vi "Example XYGraph Cursors.vi"() -> ()   [LabVIEW 2020]
uses:
  controls/CursorOptions.ctl
  Graph Extensions.lvlib
  <vilib>/ptbypt/NI_PtbyPt.lvlib
panel:
  in  "Cursor Options":T1={"font"={"Font Name"="Arial", "Size"=15, "Strikeout?"=FALSE, "Italic?"=FALSE, "Underline?"=FALSE, "Outline?"=FALSE, "Shadow?"=FALSE, "Bold?"=FALSE}, "size"=2, "Timestamp"=enum."at BOTTOM", "Vertical Line?"=TRUE, "Horizontal Line?"=TRUE, "alignment(left, top)"={"horizontal"=enum."left", "vertical"=enum."center"}, "TextFormat"=" %3$s\\n %2$.2f", "time format (%H:%M:%S)"="%I:%M:%S %p"} {"size" min=1 max=50}
  out "XY Graph":cluster{dbl[], dbl[]}[](graph)
  # "Instructions: Move the mouse over the graphs, and adjust any of the options at the right. to see the effect."
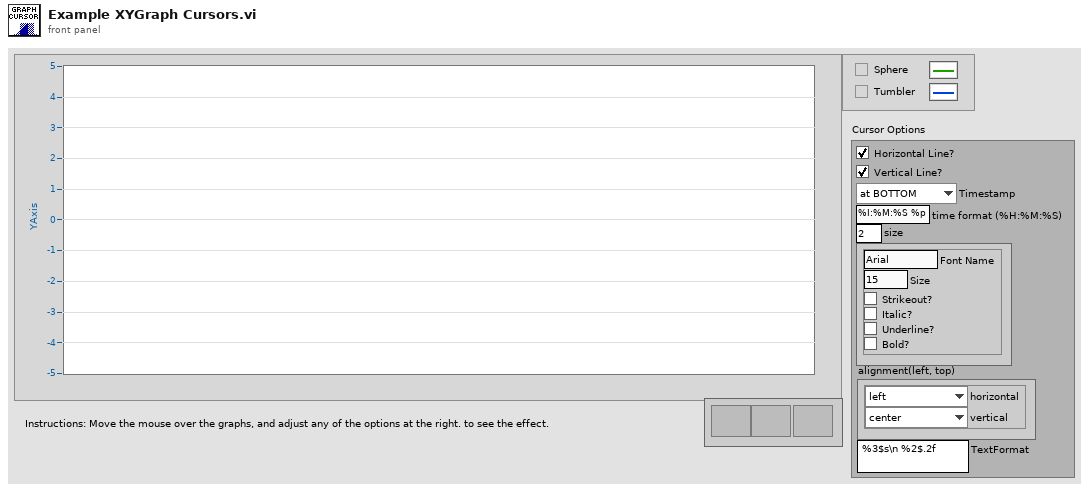
[diagram p1: front panel]
types:
  T1 = typedef "Graph Extensions.lvlib/CursorOptions.ctl" = cluster{"font":cluster{"Font Name":string, "Size":i16, "Strikeout?":bool, "Italic?":bool, "Underline?":bool, "Outline?":bool, "Shadow?":bool, "Bold?":bool}, "size":i16, "Timestamp":enum16{"at TOP", "at BOTTOM", "none"}, "Vertical Line?":bool, "Horizontal Line?":bool, "alignment(left, top)":cluster{"horizontal":enum16{"left", "center", "right"}, "vertical":enum16{"top", "center", "bottom"}}, "TextFormat":string, "time format (%H:%M:%S)":string}
  T2 = typedef "LVPoint32TypeDef.ctl" = cluster{"Horizontal":i32, "Vertical":i32}
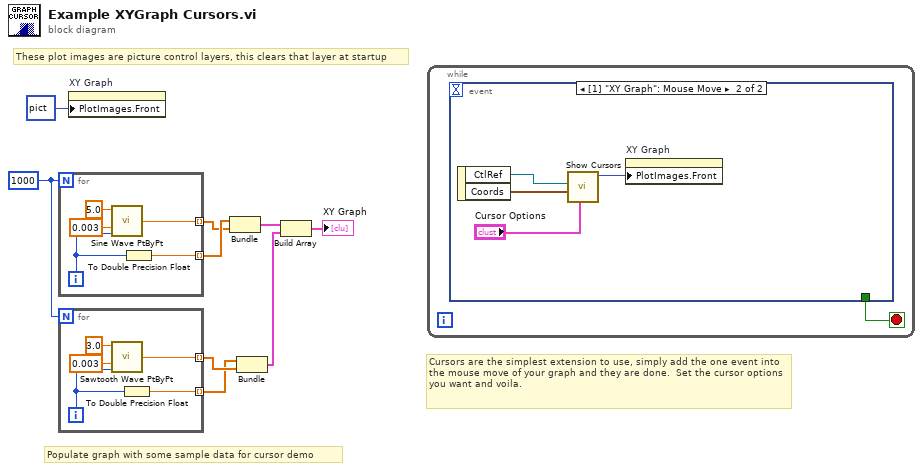
[diagram p0: block diagram]
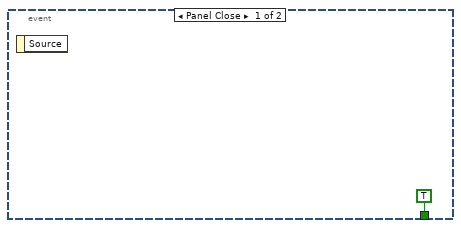
[diagram p2: hidden frame]
diagram:
  w2 = 1000
  # "These plot images are picture control layers, this clears that layer at startup"
  # "Populate graph with some sample data for cursor demo"
  # "Cursors are the simplest extension to use, simply add the one event into the mouse move of your graph and they are done.  Set the cursor options you want and voila."
  n1 = for {
    N: w2 -> [_]
    tunnel: [w14] -> w8 mode=indexing
    tunnel: [w10] -> w9 mode=indexing
    i -> [w13]
    n2 = call <vilib>:"Sine Wave PtByPt.vi"("time"=w13, "frequency"=0.003, "amplitude"=5.0) -> ("sine wave"=w14:dbl)  [unwired: 1 in]
    n3 = To Double Precision Float(number=w13) -> (double precision float=w10:dbl)
  }
  n4 = for {
    N: w2 -> [_]
    tunnel: [w19] -> w5 mode=indexing
    tunnel: [w15] -> w4 mode=indexing
    i -> [w18]
    n5 = call <vilib>:"Sawtooth Wave PtByPt.vi"("time"=w18, "frequency"=0.003, "amplitude"=3.0) -> ("sawtooth wave"=w19:dbl)  [unwired: 1 in]
    n6 = To Double Precision Float(number=w18) -> (double precision float=w15:dbl)
  }
  n7 = property on="XY Graph" class="XYGraph (strict)"("PlotImages.Front"=picture data[5B] ("Plot Images:Back")) -> ()  [unwired: 2 in, 2 out]
  n8 = Bundle(w9, w8) -> (w7:cluster{dbl[], dbl[]})  [unwired: 1 in]
  n9 = Bundle(w4, w5) -> (w3:cluster{dbl[], dbl[]})  [unwired: 1 in]
  n10 = Build Array(w7, w3) -> (→"XY Graph":cluster{dbl[], dbl[]}[])
  n11 = while {
    stop <- w20 stop-if-true
    n12 = event shown="[1] \"XY Graph\": Mouse Move" {
      selector: _ -> [_ _]
      dyn-events: _ -> [_ _]
      timeout: _ -> [_ _]
      tunnel: [TRUE _] -> w20
      event Panel Close {
        n13 = event-data() -> ()  [unwired: 1 in, 1 out]
      }
      event "XY Graph": Mouse Move {
        n14 = event-data() -> ("CtlRef"=w23:refnum<vi>, "Coords"=w25:T2)  [unwired: 1 in]
        n15 = call "Show Cursors.vi"("Cursor Options"="Cursor Options", "Coords"=w25, "XY Graph"=w23) -> ("output picture"=w22:picture)  [unwired: 7 in, 1 out]
        n16 = property on="XY Graph" class="XYGraph (strict)"("PlotImages.Front"=w22) -> ()  [unwired: 2 in, 2 out]
      }
    }
  }
